vi "Force Open New Log File Instance.vi"(8 "error in (no error)":errorcluster, 11 "Triggered Log in":refnum<class "Triggered Log.lvclass">) -> (0 "error out":errorcluster, 3 "Triggered Log out":refnum<class "Triggered Log.lvclass">)   [LabVIEW 2015, in "Triggered Log.lvclass"]
uses:
  Triggered Log.lvclass
  Triggered Log.lvclass/Triggered Log.ctl
  Engine/Classes/Logs/Segmented Logs/Segmented Log/Segmented Log.lvclass/Segmented Log.ctl
  Engine/Classes/Logs/Log Files/Log File/Log File.lvclass/Log File.ctl
  Engine/Classes/Logs/Log Files/TDMS Log File/TDMS Log File.lvclass/TDMS Log File.ctl
  Engine/Classes/Logs/Log Files/Text Log File/Text Log File.lvclass/Text Log File.ctl
  Shared/Classes/Log File Specifications/Log File Specification/Log File Specification.lvclass/Log File Specification.ctl
  Triggered Log State.ctl
  Engine/Classes/Logs/Segmented Logs/Segmented Log/Force Close Log File Instance.vi
  Engine/Classes/Logs/Segmented Logs/Segmented Log/Check Open File.vi
  On Triggered Log State Change.vi
  Engine/Classes/Triggers/Trigger/Initialize.vi
  Engine/Classes/Logs/Segmented Logs/Segmented Log/Close Log File Instance.vi
  Engine/Classes/Logs/Segmented Logs/Segmented Log/Open Log File Instance.vi
  Engine/Classes/Triggers/Digital Edge Trigger/Initialize Digital Edge Trigger.vi
  Engine/Classes/Triggers/Analog Edge Trigger/Initialize Analog Edge Trigger.vi
  Engine/Classes/Triggers/Value Change Trigger/Initialize Value Change Trigger.vi
  Engine/Classes/Logs/Log Files/Log File/Close Log File.vi
  Engine/Classes/Logs/Segmented Logs/Segmented Log/Make File Read-Only.vi
  Engine/Classes/Logs/Segmented Logs/Segmented Log/On Segmented Log Complete.vi
  Engine/Classes/Logs/Segmented Logs/Segmented Log/On File Close.vi
  Shared/Classes/Log File Specifications/Log File Specification/Open Log File.vi
  Shared/Classes/Log File Specifications/Log File Specification/Set Path Tag.vi
  Engine/Classes/Logs/Segmented Logs/Segmented Log/On File Open.vi
  Shared/Classes/Log File Specifications/Log File Specification/Set Filename Offset.vi
  Engine/Classes/Logs/Log Files/TDMS Log File/Close TDMS Log File.vi
  Engine/Classes/Logs/Log Files/Text Log File/Close Text Log File.vi
  Shared/Classes/Log File Specifications/Log File Specification/Build File Path.vi
  Shared/Classes/Log File Specifications/Log File Specification/Resolve File Conflicts.vi
  Engine/Classes/Triggers/Trigger/Finalize.vi
  <vilib>/Utility/error.llb/Error Cluster From Error Code.vi
  Shared/Classes/Log File Specifications/Log File Specification/Initialize Log File.vi
  <vilib>/Utility/libraryn.llb/Create Directory Recursive.vi
  <vilib>/Utility/libraryn.llb/Check if File or Folder Exists.vi
  <vilib>/Utility/libraryn.llb/Get File Extension.vi
  Engine/Classes/Triggers/Value Change Trigger/Value Change Trigger.lvclass
  Engine/Classes/Triggers/Analog Edge Trigger/Analog Edge Trigger.lvclass
  Engine/Classes/Triggers/Digital Edge Trigger/Digital Edge Trigger.lvclass
  Engine/Classes/Logs/Log Files/Log File/Log File.lvclass
  Engine/Classes/Logs/Log Files/Text Log File/Text Log File.lvclass
  Engine/Classes/Logs/Log Files/TDMS Log File/TDMS Log File.lvclass
  Engine/Classes/Logs/Segmented Logs/Segmented Log/Segmented Log.lvclass
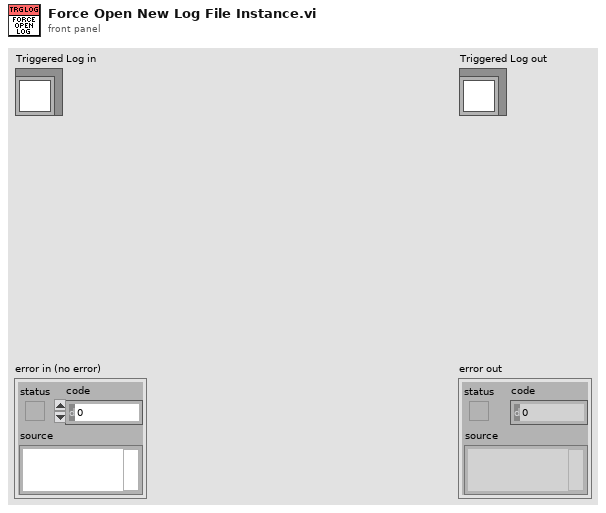
[diagram p1: front panel]
types:
  T1 = typedef "Triggered Log.lvclass/Triggered Log State.ctl" = enum16{"Waiting on Trigger", "Triggered", "Posttrigger", "Complete", "Idle", "Error"}
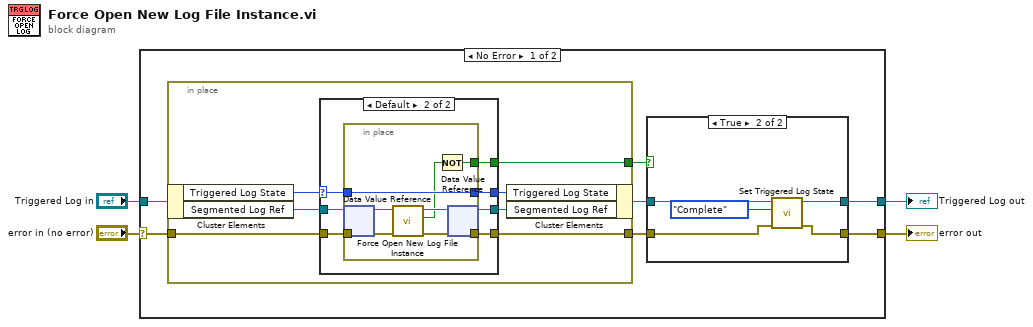
[diagram p0: block diagram]
diagram:
  n1 = case shown="No Error" "error in (no error)" {
    selector: "error in (no error)" -> [w10 w44]
    tunnel: [w6 w44] -> w3
    tunnel: [w7 w43] -> w1
    tunnel: "Triggered Log in" -> [w11 w43]
    frame No Error {
      n2 = in-place {
        in-place-border: w10 -> [w24]
        in-place-border: [w23] -> w9
        in-place-border: [w19] -> w5
        n3 = in-place-cluster #1(w11) -> ("Triggered Log State"=w20:T1, "Segmented Log Ref"=w25:refnum<data-value>)
        n4 = case shown="Default" w20 {
          selector: w20 -> [w28 w30]
          tunnel: w25 -> [w27 w35]
          tunnel: w24 -> [w26 w34]
          tunnel: [w26 w33] -> w23
          tunnel: [w28 w32] -> w22
          tunnel: [w27 w31] -> w21
          tunnel: [_ w29] -> w19
          frame "Complete" {
          }
          frame Default {
            n5 = in-place {
              in-place-border: w34 -> [w41]
              in-place-border: [w40] -> w33
              in-place-border: w30 -> [w38]
              in-place-border: [w38] -> w32
              in-place-border: [w36] -> w29
              n6 = in-place-dvr #2(w35) -> (w42:refnum<class "Segmented Log.lvclass">)  [unwired: 1 out]
              n7 = call "Force Open New Log File Instance.vi"("error in (no error)"=w41, "Segmented Log in"=w42) -> ("error out"=w40:errorcluster, "Log Active"=w37:bool, "Segmented Log out"=w39:refnum<class "Segmented Log.lvclass">)  [unwired: 7 in]
              n8 = Not(x=w37) -> (.not. x?=w36:bool)
              n9 = in-place-dvr #2(w39) -> (w31:refnum<data-value>)  [unwired: 1 out]
            }
          }
        }
        n10 = in-place-cluster #1("Triggered Log State"=w22, "Segmented Log Ref"=w21) -> (w8:refnum<class "Triggered Log.lvclass">)
      }
      n11 = case shown="True" w5 {
        tunnel: w9 -> [w12 w18]
        tunnel: [w12 w17] -> w6
        tunnel: [w13 w16] -> w7
        tunnel: w8 -> [w13 w15]
        frame False {
        }
        frame True {
          n12 = call "Set Triggered Log State.vi"("error in (no error)"=w18, "Triggered Log State"=Triggered_Log_State."Complete", "Triggered Log in"=w15) -> ("error out"=w17:errorcluster, "Triggered Log out"=w16:refnum<class "Triggered Log.lvclass">)  [unwired: 7 in]
        }
      }
    }
    frame Error {
    }
  }
  "error out" <- w3
  "Triggered Log out" <- w1
